vi "tcpServerStateMachine.vi"(8 "error in (no error)":errorcluster, 11 "TcpServerTel in":refnum<class "TcpServerTel.lvclass">) -> (0 "error out":errorcluster, 3 "TcpServerTel out":refnum<class "TcpServerTel.lvclass">)   [LabVIEW 2018, in "TcpServerTel.lvclass"]
doc: "TCP Server State Machine. Put the VI in preallocated reentrant clone execution.\n\nStates:\n\n1.- Create Listener.\n2.- Wait on Listener.\n3.- Read TCP Packet.\n4.- Close Connection.\n5.- Stop Server."
uses:
  TcpServerTel.lvclass
  home/pcortes/Documents/github/ts_labview_tcp_json/src/TcpServerBase/TcpServerBase.lvclass
  TcpServerBase/TcpServerBase.lvclass/TcpServerBase.ctl
  TcpServerBase/typedef/tcpConnectionTypeDef.ctl
  TcpServerBase/TcpServerBase.lvclass
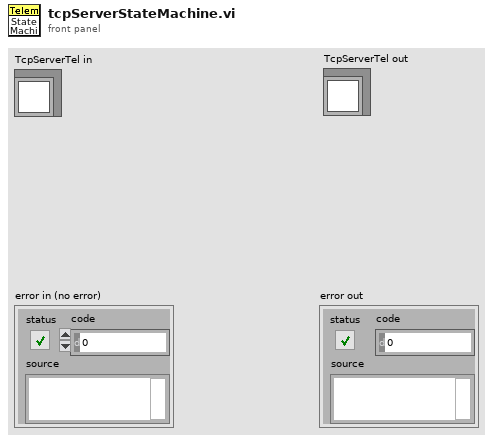
[diagram p1: front panel]
types:
  T1 = typedef "TcpServerBase.lvclass/tcpConnectionTypeDef.ctl" = cluster{"connection ID":refnum<k5>, "firstConnection":bool}
  T2 = enum16{"Standard", "Buffered", "CRLF", "Immediate"}
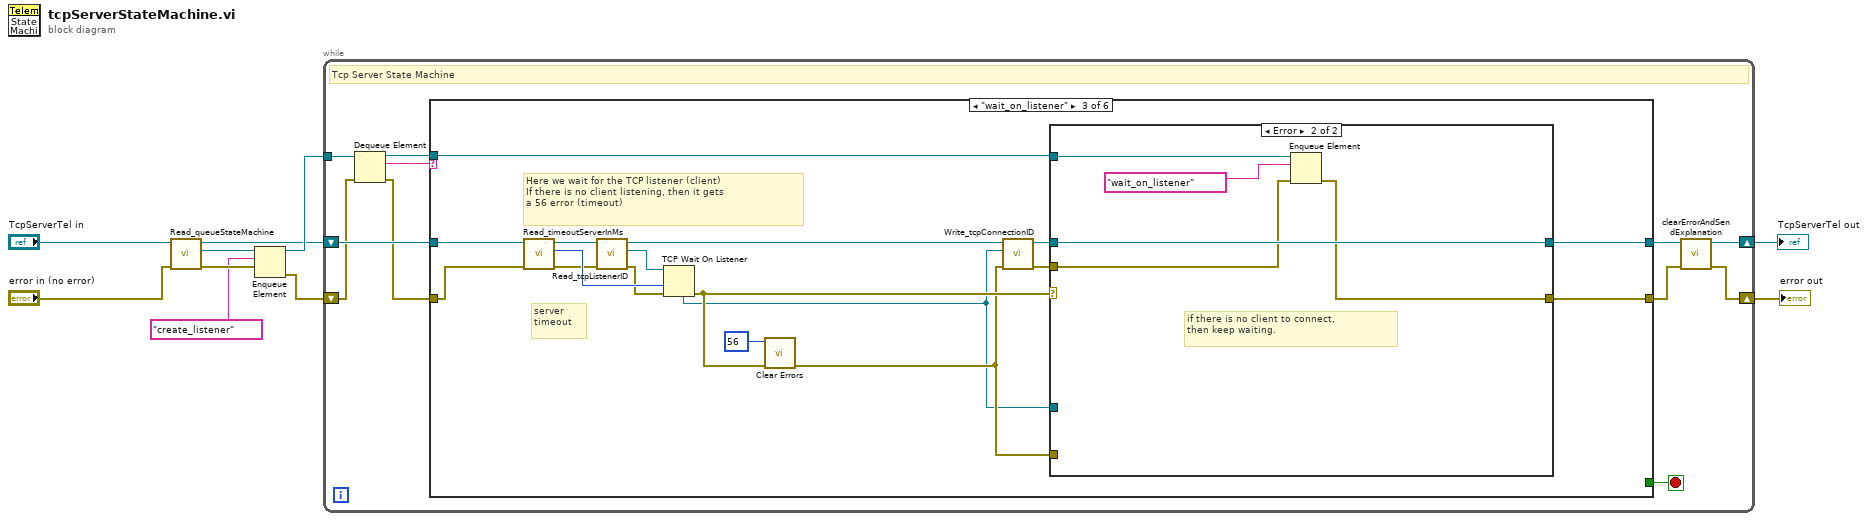
[diagram p0: block diagram]
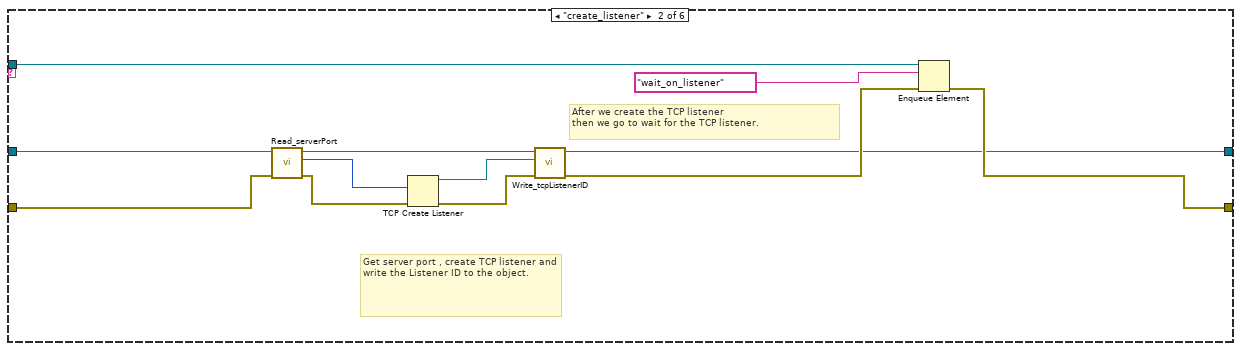
[diagram p3: hidden frame]
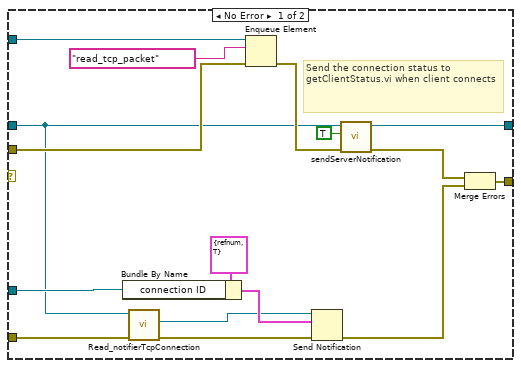
[diagram p4: hidden frame]
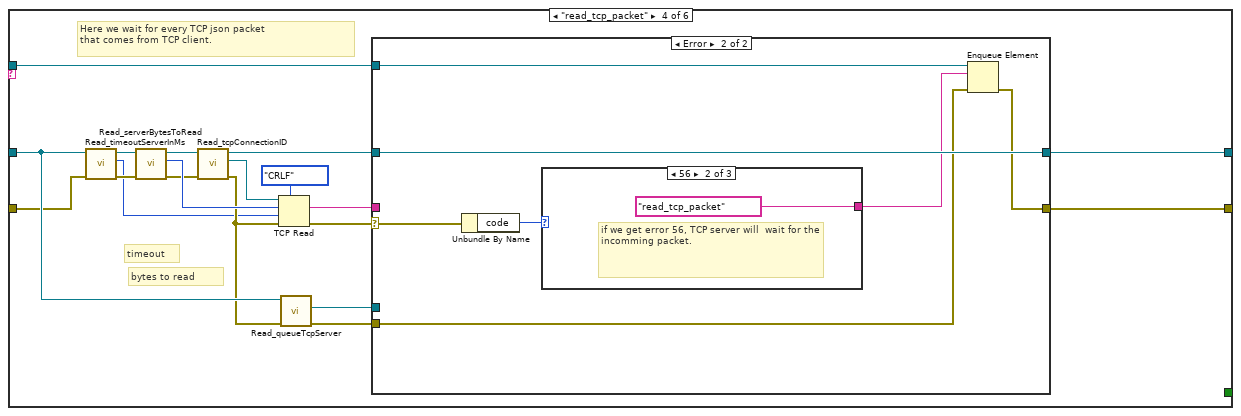
[diagram p5: hidden frame]
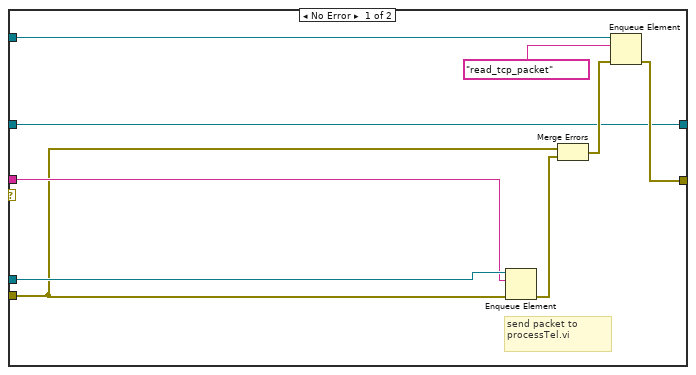
[diagram p6: hidden frame]
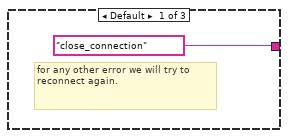
[diagram p7: hidden frame]
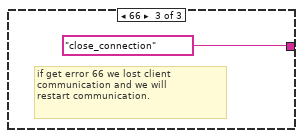
[diagram p8: hidden frame]
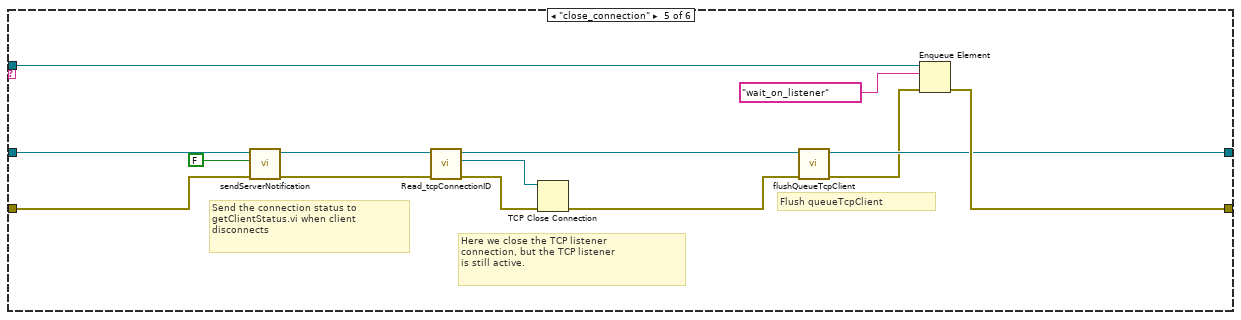
[diagram p9: hidden frame]
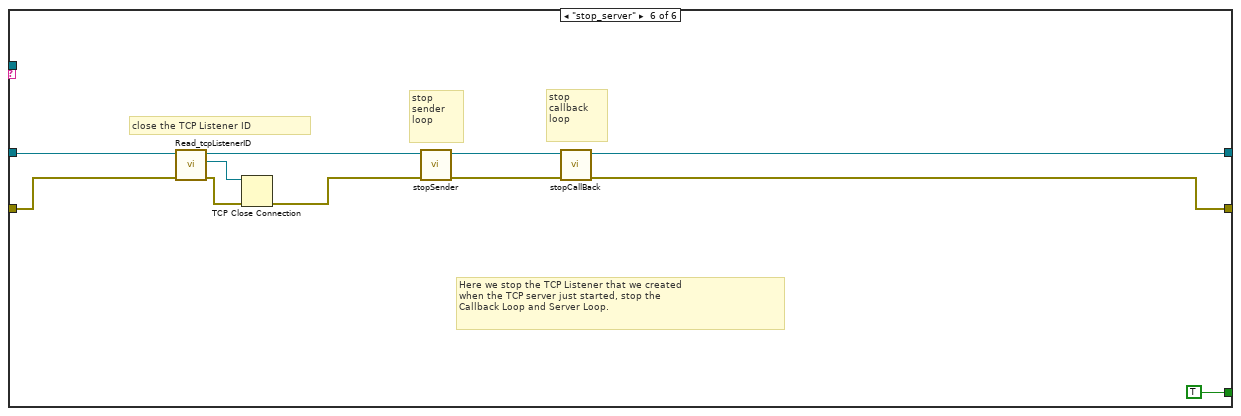
[diagram p10: hidden frame]
diagram:
  n1 = call "Read_queueStateMachine.vi"("error in (no error)"="error in (no error)", "TcpServerBase in"="TcpServerTel in") -> ("error out"=w5:errorcluster, "queueStateMachine"=w6:refnum<queue>, "TcpServerBase out"=w1:refnum<class "TcpServerTel.lvclass">)  [unwired: 7 in]
  n2 = Enqueue Element(queue=w6, element="create_listener", error in (no error)=w5) -> (queue out=w3:refnum<queue>, error out=w2:errorcluster)  [unwired: 1 in, 1 out]
  n3 = while {
    shift-right: [w12] -> w9
    shift-left: w1 -> [w21]
    shift-right: [w14] -> w10
    shift-left: w2 -> [w16]
    tunnel: w3 -> [w11]
    stop <- w18 stop-if-true
    # "Tcp Server State Machine"
    n4 = Dequeue Element(queue=w11, error in (no error)=w16) -> (queue out=w20:refnum<queue>, element=w19:string, error out=w15:errorcluster)  [unwired: 1 in, 1 out]
    n5 = case shown="\"wait_on_listener\"" w19 {
      tunnel: w21 -> [w23 w33 w49 w87 w117 w134]
      tunnel: [w23 w24 w48 w84 w112 w125] -> w13
      tunnel: w20 -> [_ w29 w47 w78 w124 _]
      tunnel: [_ _ _ _ _ TRUE] -> w18
      tunnel: w15 -> [w22 w27 w45 w82 w121 w131]
      tunnel: [w22 w25 w39 w77 w119 w127] -> w17
      frame Default {
        # "Do notihig for now."
      }
      frame "create_listener" {
        # "After we create the TCP listener\nthen we go to wait for the TCP listener."
        # "Get server port , create TCP listener and write the Listener ID to the object."
        n6 = call "Read_serverPort.vi"("error in (no error)"=w27, "TcpServerBase in"=w33) -> ("error out"=w34:errorcluster, "serverPort"=w35:u16, "TcpServerBase out"=w32:refnum<class "TcpServerTel.lvclass">)  [unwired: 7 in]
        n7 = TCP Create Listener(8:w34, 10:w35) -> (0:w30:errorcluster, 3:w31:refnum<k5>)  [unwired: 3 in, 1 out]
        n8 = call "Write_tcpListenerID.vi"("error in (no error)"=w30, "tcpListenerID"=w31, "TcpServerBase in"=w32) -> ("error out"=w26:errorcluster, "TcpServerBase out"=w24:refnum<class "TcpServerTel.lvclass">)  [unwired: 7 in]
        n9 = Enqueue Element(queue=w29, element="wait_on_listener", error in (no error)=w26) -> (error out=w25:errorcluster)  [unwired: 1 in, 2 out]
      }
      frame "wait_on_listener" {
        # "Here we wait for the TCP listener (client)\nIf there is no client listening, then it gets\na 56 error (timeout)"
        # "server\ntimeout"
        n10 = call "Read_timeoutServerInMs.vi"("error in (no error)"=w45, "TcpServerBase in"=w49) -> ("error out"=w44:errorcluster, "timeoutServerInMs"=w50:i32, "TcpServerBase out"=w51:refnum<class "TcpServerTel.lvclass">)  [unwired: 7 in]
        n11 = call "Read_tcpListenerID.vi"("error in (no error)"=w44, "TcpServerBase in"=w51) -> ("error out"=w43:errorcluster, "tcpListenerID"=w52:refnum<k5>, "TcpServerBase out"=w38:refnum<class "TcpServerTel.lvclass">)  [unwired: 7 in]
        n12 = TCP Wait On Listener(8:w43, 9:w50, 11:w52) -> (0:w41:errorcluster, 4:w36:refnum<k5>)  [unwired: 1 in, 3 out]
        n13 = call <vilib>:"Clear Errors.vi"("error in (no error)"=w41, "specific error code to clear (0: all)"=56) -> ("error out"=w37:errorcluster)  [unwired: 4 in, 1 out]
        n14 = call "Write_tcpConnectionID.vi"("error in (no error)"=w37, "tcpConnectionID"=w36, "TcpServerBase in"=w38) -> ("error out"=w40:errorcluster, "TcpServerBase out"=w46:refnum<class "TcpServerTel.lvclass">)  [unwired: 7 in]
        n15 = case shown="Error" w41 {
          tunnel: w46 -> [w56 w73]
          tunnel: [w58 w73] -> w48
          tunnel: w47 -> [w67 w72]
          tunnel: w40 -> [w66 w70]
          tunnel: [w61 w69] -> w39
          tunnel: w37 -> [w55 _]
          tunnel: w36 -> [w62 _]
          frame No Error {
            # "Send the connection status to getClientStatus.vi when client connects"
            n16 = Bundle By Name(cluster=T1 {"connection ID"=refnum, "firstConnection"=TRUE} ("TcpConnectionCluster"), "connection ID"=w62) -> (w64:T1)
            n17 = call "Read_notifierTcpConnection.vi"("error in (no error)"=w55, "TcpServerBase in"=w56) -> ("error out"=w54:errorcluster, "notifierTcpConnection"=w53:refnum<notifier>)  [unwired: 7 in, 1 out]
            n18 = Enqueue Element(queue=w67, element="read_tcp_packet", error in (no error)=w66) -> (error out=w65:errorcluster)  [unwired: 1 in, 2 out]
            n19 = Send Notification(notification=w64, notifier=w53, error in (no error)=w54) -> (error out=w60:errorcluster)  [unwired: 1 out]
            n20 = call "sendServerNotification.vi"("error in (no error)"=w65, "connectionStatus"=TRUE ("serverStatus"), "TcpServerBase in"=w56) -> ("error out"=w59:errorcluster, "TcpServerBase out"=w58:refnum<class "TcpServerTel.lvclass">)  [unwired: 7 in]
            n21 = Merge Errors(w59, w60) -> (w61:errorcluster)
          }
          frame Error {
            # "if there is no client to connect, \nthen keep waiting."
            n22 = Enqueue Element(queue=w72, element="wait_on_listener", error in (no error)=w70) -> (error out=w69:errorcluster)  [unwired: 1 in, 2 out]
          }
        }
      }
      frame "read_tcp_packet" {
        # "timeout"
        # "Here we wait for every TCP json packet\nthat comes from TCP client."
        # "bytes to read"
        n23 = call "Read_timeoutServerInMs.vi"("TcpServerBase in"=w87) -> ("timeoutServerInMs"=w74:i32, "TcpServerBase out"=w75:refnum<class "TcpServerTel.lvclass">)  [unwired: 8 in, 1 out]
        n24 = call "Read_serverBytesToRead.vi"("error in (no error)"=w82, "TcpServerBase in"=w75) -> ("error out"=w83:errorcluster, "serverBytesToRead"=w88:i32, "TcpServerBase out"=w86:refnum<class "TcpServerTel.lvclass">)  [unwired: 7 in]
        n25 = call "Read_tcpConnectionID.vi"("error in (no error)"=w83, "TcpServerBase in"=w86) -> ("error out"=w80:errorcluster, "tcpConnectionID"=w76:refnum<k5>, "TcpServerBase out"=w85:refnum<class "TcpServerTel.lvclass">)  [unwired: 7 in]
        n26 = TCP Read(connection ID=w76, bytes to read=w88, error in (no error)=w80, 7:T2."CRLF" ("mode (standard)"), 9:w74) -> (data out=w91:string, error out=w89:errorcluster)  [unwired: 1 out]
        n27 = call "Read_queueTcpServer.vi"("error in (no error)"=w80, "TcpServerBase in"=w87) -> ("error out"=w79:errorcluster, "queueTcpServer"=w81:refnum<queue>)  [unwired: 7 in, 1 out]
        n28 = case shown="Error" w89 {
          selector: w89 -> [_ w107]
          tunnel: w91 -> [w99 _]
          tunnel: w81 -> [w100 _]
          tunnel: w85 -> [w93 w105]
          tunnel: [w93 w105] -> w84
          tunnel: w79 -> [w92 w102]
          tunnel: w78 -> [w98 w104]
          tunnel: [w96 w101] -> w77
          frame No Error {
            # "send packet to\nprocessTel.vi"
            n29 = Enqueue Element(queue=w100, element=w99, error in (no error)=w92) -> (error out=w95:errorcluster)  [unwired: 1 in, 2 out]
            n30 = Merge Errors(w92, w95) -> (w94:errorcluster)
            n31 = Enqueue Element(queue=w98, element="read_tcp_packet", error in (no error)=w94) -> (error out=w96:errorcluster)  [unwired: 1 in, 2 out]
          }
          frame Error {
            n32 = Unbundle By Name(w107) -> ("code"=w106:i32)
            n33 = case shown="56" w106 {
              tunnel: ["close_connection" "read_tcp_packet" "close_connection"] -> w103
              frame Default {
                # "for any other error we will try to reconnect again."
              }
              frame 56 {
                # "if we get error 56, TCP server will  wait for the incomming packet."
              }
              frame 66 {
                # "if get error 66 we lost client \ncommunication and we will\nrestart communication."
              }
            }
            n34 = Enqueue Element(queue=w104, element=w103, error in (no error)=w102) -> (error out=w101:errorcluster)  [unwired: 1 in, 2 out]
          }
        }
      }
      frame "close_connection" {
        # "Flush queueTcpClient"
        # "Send the connection status to getClientStatus.vi when client disconnects"
        # "Here we close the TCP listener\nconnection, but the TCP listener\nis still active."
        n35 = call "sendServerNotification.vi"("error in (no error)"=w121, "connectionStatus"=FALSE ("serverStatus"), "TcpServerBase in"=w117) -> ("error out"=w118:errorcluster, "TcpServerBase out"=w116:refnum<class "TcpServerTel.lvclass">)  [unwired: 7 in]
        n36 = call "Read_tcpConnectionID.vi"("error in (no error)"=w118, "TcpServerBase in"=w116) -> ("error out"=w120:errorcluster, "tcpConnectionID"=w122:refnum<k5>, "TcpServerBase out"=w114:refnum<class "TcpServerTel.lvclass">)  [unwired: 7 in]
        n37 = TCP Close Connection(connection ID=w122, error in (no error)=w120) -> (error out=w113:errorcluster)  [unwired: 1 in, 1 out]
        n38 = call "flushQueueTcpClient.vi"("error in (no error)"=w113, "TcpServerBase in"=w114) -> ("error out"=w111:errorcluster, "TcpServerBase out"=w112:refnum<class "TcpServerTel.lvclass">)  [unwired: 8 in]
        n39 = Enqueue Element(queue=w124, element="wait_on_listener", error in (no error)=w111) -> (error out=w119:errorcluster)  [unwired: 1 in, 2 out]
      }
      frame "stop_server" {
        # "Here we stop the TCP Listener that we created\nwhen the TCP server just started, stop the \nCallback Loop and Server Loop."
        # "close the TCP Listener ID"
        # "stop\nsender\nloop"
        # "stop\ncallback\nloop"
        n40 = call "Read_tcpListenerID.vi"("error in (no error)"=w131, "TcpServerBase in"=w134) -> ("error out"=w130:errorcluster, "tcpListenerID"=w135:refnum<k5>, "TcpServerBase out"=w126:refnum<class "TcpServerTel.lvclass">)  [unwired: 7 in]
        n41 = TCP Close Connection(connection ID=w135, error in (no error)=w130) -> (error out=w129:errorcluster)  [unwired: 1 in, 1 out]
        n42 = call "stopSender.vi"("error in (no error)"=w129, "TcpServerBase in"=w126) -> ("error out"=w128:errorcluster, "TcpServerBase out"=w132:refnum<class "TcpServerTel.lvclass">)  [unwired: 8 in]
        n43 = call "stopCallBack.vi"("error in (no error)"=w128, "TcpServerBase in"=w132) -> ("error out"=w127:errorcluster, "TcpServerBase out"=w125:refnum<class "TcpServerTel.lvclass">)  [unwired: 8 in]
      }
    }
    n44 = call "clearErrorAndSendExplanation.vi"("error in (no error)"=w17, "TcpServerBase in"=w13) -> ("error out"=w14:errorcluster, "TcpServerBase out"=w12:refnum<class "TcpServerTel.lvclass">)  [unwired: 8 in]
  }
  "error out" <- w10
  "TcpServerTel out" <- w9
